vi "write-image-name-script-2017.vi"(0 "Image Name Input":string="image00000.tif", 11 "Error in":errorcluster) -> (4 "result string from input file after new insertion":string, 15 "Error out":errorcluster)   [LabVIEW 2017]
doc: "VI devoloped at University of Twente, BioPhysical Engineering, used for running ImageJ in LabVIEW. Insert the macro to be run in the top string. Make sure the macro is in the C:\\Program Files\\ImageJ directory."
panel:
  out "New scrip file":string
  out "Input String from script":string
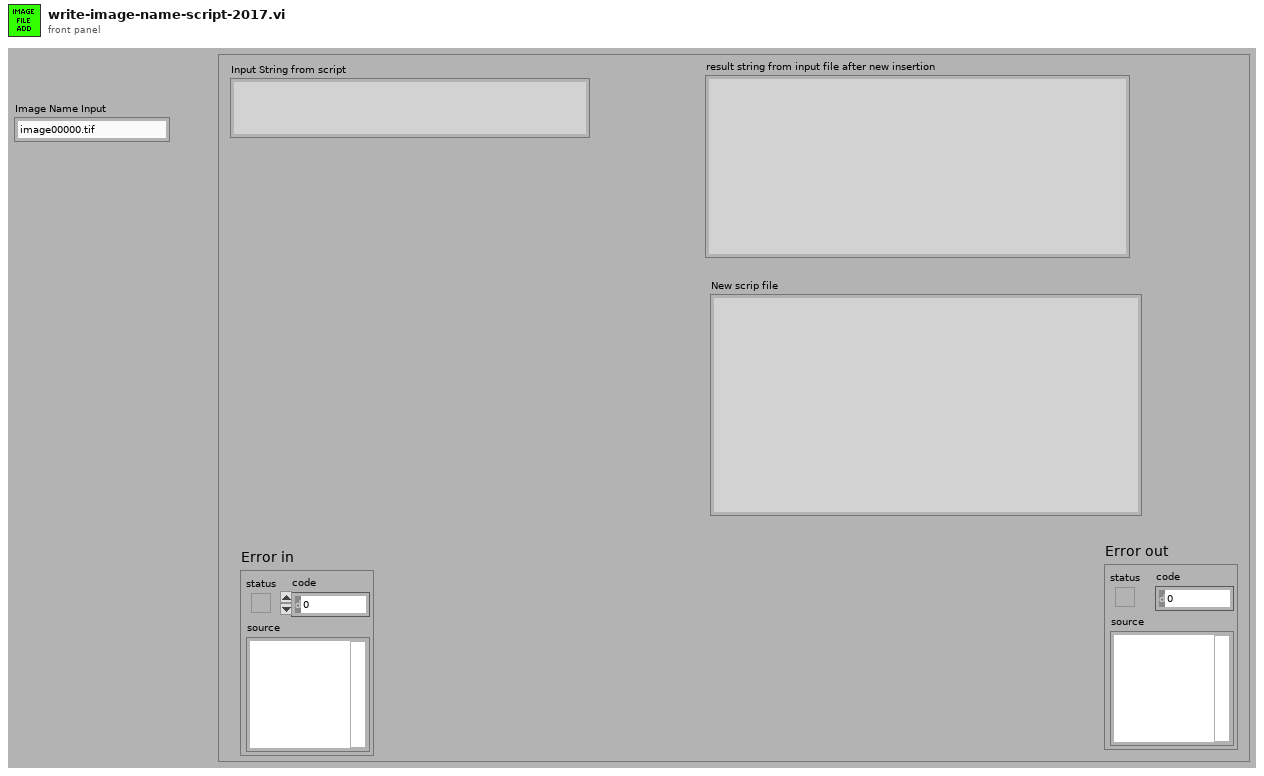
[diagram p1: front panel]
types:
  T1 = enum16{"open", "replace", "create", "open or create", "replace or create", "replace or create with confirmation"}
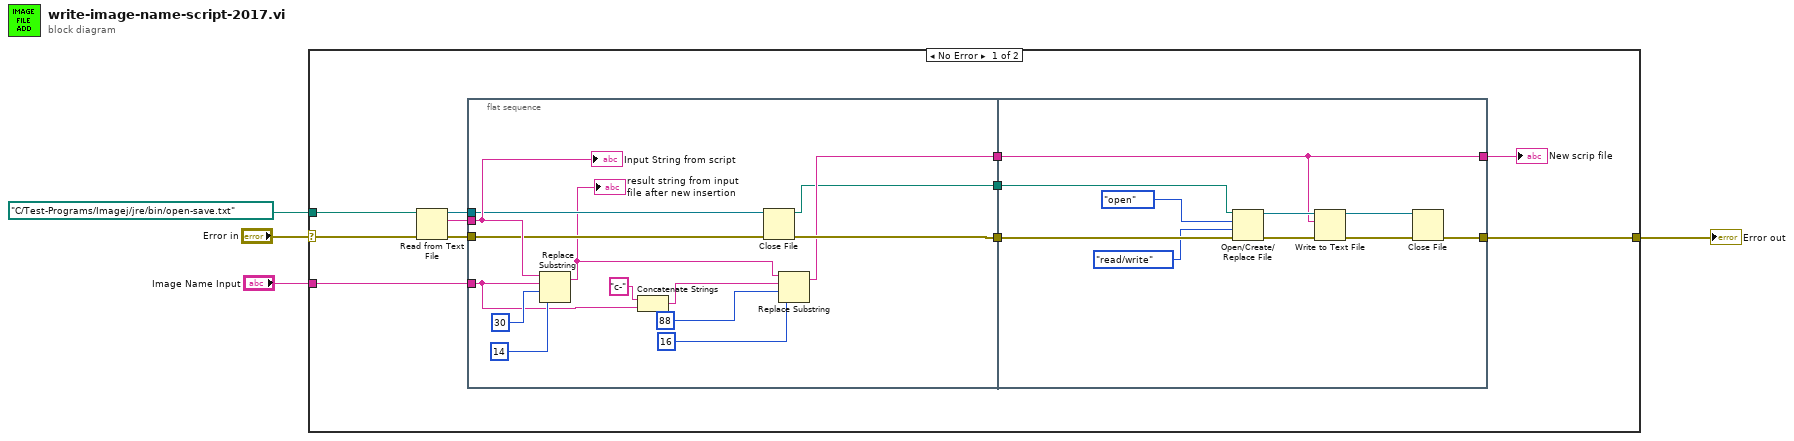
[diagram p0: block diagram]
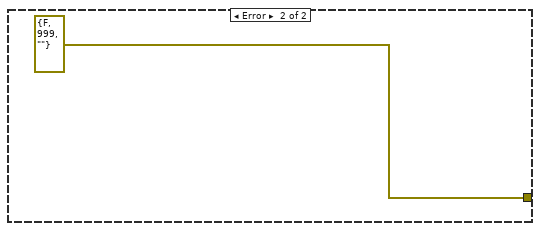
[diagram p2: hidden frame]
diagram:
  n1 = case shown="No Error" "Error in" {
    selector: "Error in" -> [w15 _]
    tunnel: [w6 errorcluster {"status"=FALSE, "code"=999, "source"=""} ("error out")] -> w3
    tunnel: path "C:/Test-Programs/Imagej/jre/bin/open-save.txt" ("file (use dialog)") -> [w11 _]
    tunnel: "Image Name Input" -> [w13 _]
    frame No Error {
      n2 = Read from Text File(file (use dialog)=w11, error in=w15) -> (refnum out=w10:refnum<file>, text=w14:string, error out=w12:errorcluster)  [unwired: 2 in, 1 out]
      n3 = flat-sequence {
        tunnel: w14 -> [w29]
        tunnel: w13 -> [w22]
        tunnel: w12 -> [w21]
        tunnel: w10 -> [w19]
        tunnel: [w20] -> w9
        tunnel: [w18] -> w8
        tunnel: [w16] -> w5
        tunnel: w9 -> [w39]
        tunnel: w8 -> [w34]
        tunnel: [w34] -> w7
        tunnel: [w31] -> w6
        tunnel: w5 -> [w30]
        frame #0 {
          n4 = Replace Substring(2:14 ("length (len. of substring)"), 3:30 ("offset (0)"), 4:w22, 5:w29) -> (1:w17:string)  [unwired: 1 out]
          "result string from input file after new insertion" <- w17
          n5 = Concatenate Strings("c-" ("string"), w22) -> (w24:string)
          n6 = Close File(refnum=w19, error in=w21) -> (path=w16:path, error out=w20:errorcluster)
          n7 = Replace Substring(2:16 ("length (len. of substring)"), 3:88 ("offset (0)"), 4:w24, 5:w17) -> (1:w18:string)  [unwired: 1 out]
          "Input String from script" <- w29
        }
        frame #1 {
          n8 = Open/Create/Replace File(file path (use dialog)=w30, error in=w39, operation (0:open)=T1."open", access (0:read/write)=enum16{"read/write", "read-only", "write-only"}."read/write") -> (refnum out=w35:refnum<file>, error out=w36:errorcluster)  [unwired: 2 in, 1 out]
          n9 = Write to Text File(file (use dialog)=w35, text=w34, error in=w36) -> (refnum out=w32:refnum<file>, error out=w33:errorcluster)  [unwired: 1 in, 1 out]
          n10 = Close File(refnum=w32, error in=w33) -> (error out=w31:errorcluster)  [unwired: 1 out]
        }
      }
      "New scrip file" <- w7
    }
    frame Error {
    }
  }
  "Error out" <- w3
